vi "读取命令发送.vi"(1 "数值":dbl) -> ()   [LabVIEW 2018]
panel:
  in  "要发送的数据":string[][](table)
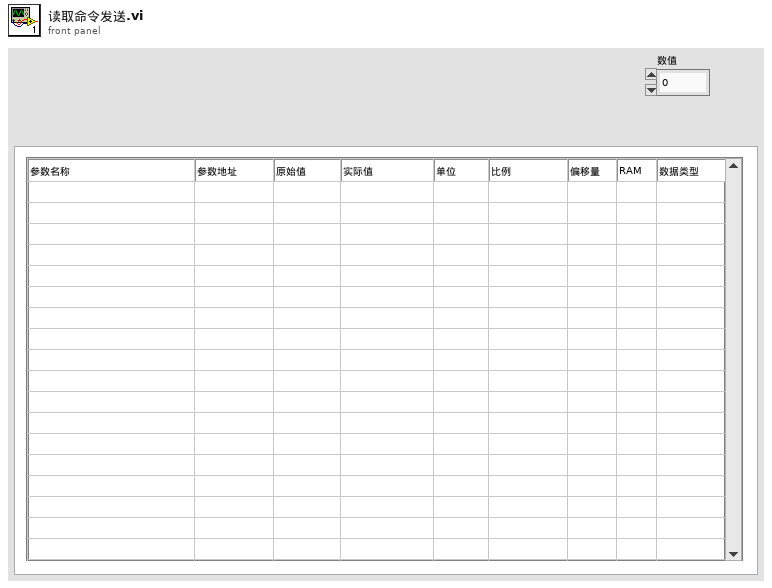
[diagram p1: front panel]
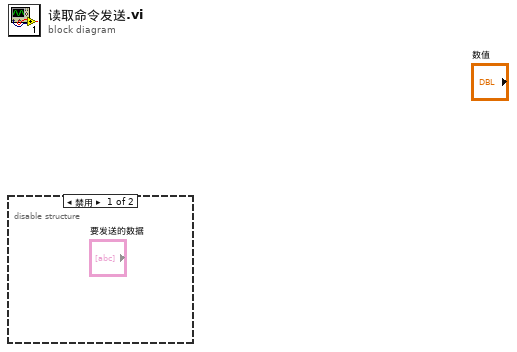
[diagram p0: block diagram]
diagram:
  n1 = disable-structure shown="禁用" {
    frame Disabled {
    }
    frame Enabled {
    }
  }
